vi "QMOLEdll.vi"(8 "error in (no error)":errorcluster, 11 "Inputs":cluster{"qkg":dbl, "xlkg":dbl, "xvkg":dbl}) -> (0 "error out":errorcluster, 3 "Outputs":T1)   [LabVIEW 2016]
doc: "subroutine QMOLEdll(qkg, xlkg, xvkg, qmol, x, y, wliq, wvap, ierr, herr, herr_length\n\nConverts quality and composition on a mass basis to a molar basis\n\nINPUTS:\nqkg -- Quality on mass basis (mass of vapor/total mass) qkg = 0 indicates saturated\n liquid qkg = 1 indicates saturated vapor 0 < qkg < 1 indicates a two-phase state qkg <\n 0 or qkg > 1 are not allowed and will result in warning\nxlkg -- mass composition of liquid phase [array of mass frac]\nxvkg -- mass composition of vapor phase [array of mass frac]\n\nOUTPUTS:\nqmol -- quality on mass basis [mass of vapor/total mass]\nx -- molar composition of liquid phase [array of mol frac]\ny -- molar composition of vapor phase [array of mol frac]\nwliq -- molecular weight of liquid phase [g/mol]\nwvap -- molecular weight of vapor phase [g/mol]\nierr -- error flag: 0 = all inputs within limits, -19 = input q < 0 or > 1\nherr -- error string (character*255 variable if ierr<>0)\nherr_length --length of variable herr (default: 255)"
uses:
  REFPROP.DLL
panel:
  # "REFPROP-QMOLEdll.vi"
  # "void  QMOLEdll(double *qkg, double *xlkg, double *xvkg, double *qmol, double *x, double *y, double *wliq, double *wvap, int32_t *ierr, CStr herr, int32_t herr_length)"
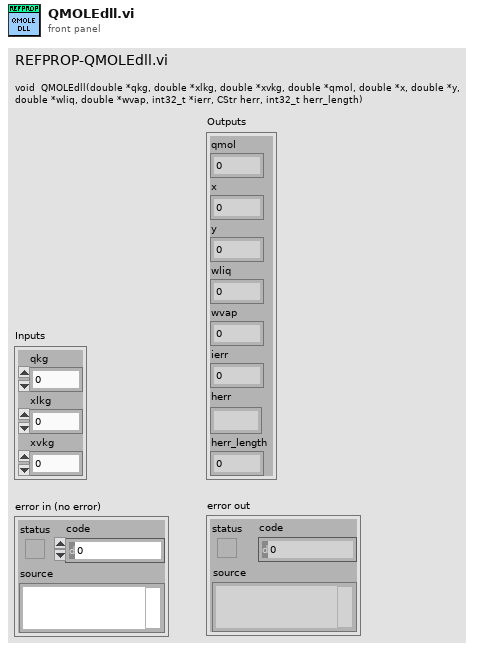
[diagram p1: front panel]
types:
  T1 = cluster{"qmol":dbl, "x":dbl, "y":dbl, "wliq":dbl, "wvap":dbl, "ierr":i32, "herr":string, "herr_length":i32}
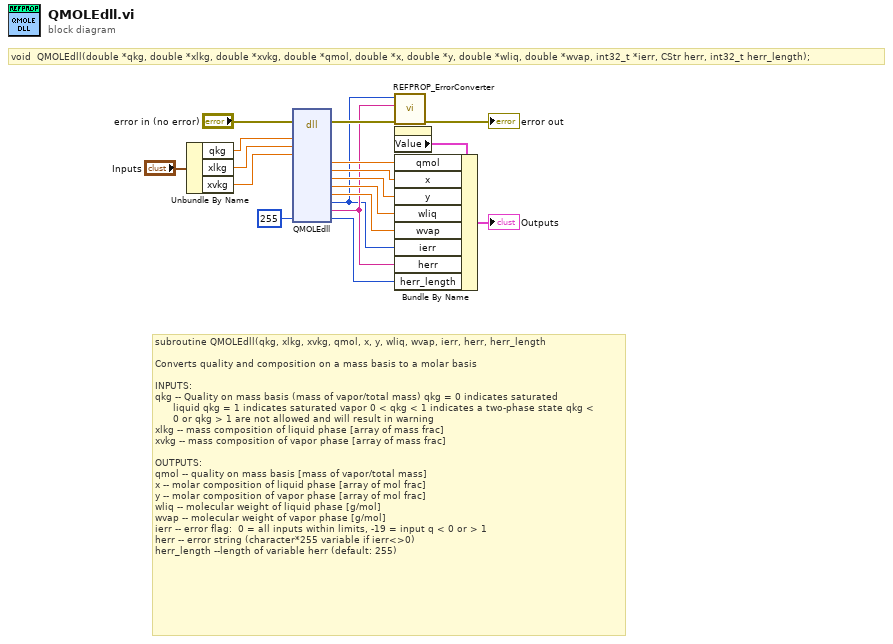
[diagram p0: block diagram]
diagram:
  # "void  QMOLEdll(double *qkg, double *xlkg, double *xvkg, double *qmol, double *x, double *y, double *wliq, double *wvap, int32_t *ierr, CStr herr, int32_t herr_length);"
  # "subroutine QMOLEdll(qkg, xlkg, xvkg, qmol, x, y, wliq, wvap, ierr, herr, herr_length\n\nConverts quality and composition on a mass basis to a molar basis\n\nINPUTS:\nqkg -- Quality on mass basis (mass of vapor/total mass) qkg = 0 indicates saturated\n      liquid qkg = 1 indicates saturated vapor 0 < qkg < 1 indicates a two-phase state qkg <\n      0 or qkg > 1 are not allowed and will result in warning\nxlkg -- mass composition of liquid phase [array of mass frac]\nxvkg -- mass composition of vapor phase [array of mass frac]\n\nOUTPUTS:\nqmol -- quality on mass basis [mass of vapor/total mass]\nx -- molar composition of liquid phase [array of mol frac]\ny -- molar composition of vapor phase [array of mol frac]\nwliq -- molecular weight of liquid phase [g/mol]\nwvap -- molecular weight of vapor phase [g/mol]\nierr -- error flag:  0 = all inputs within limits, -19 = input q < 0 or > 1\nherr -- error string (character*255 variable if ierr<>0)\nherr_length --length of variable herr (default: 255)"
  n1 = Unbundle By Name("Inputs") -> ("qkg"=w13:dbl, "xlkg"=w12:dbl, "xvkg"=w11:dbl)
  n2 = dll-call lib="S:/009 - Testing/02 - Performance Testing/REFPROP/REFPROP.*" fn="QMOLEdll"(error in="error in (no error)", "qkg"=w13, "xlkg"=w12, "xvkg"=w11, "herr_length"=255 ("ln")) -> (error out=w17:errorcluster, "qmol"=w3:dbl, "x"=w4:dbl, "y"=w5:dbl, "wliq"=w6:dbl, "wvap"=w7:dbl, "ierr"=w1:i32, "herr"=w2:string, "herr_length"=w8:i32)  [unwired: 13 in, 1 out]
  n3 = call "REFPROP_ErrorConverter.vi"("error in (no error)"=w17, "Error Message"=w2, "Error Code"=w1) -> ("error out"=→"error out":errorcluster)  [unwired: 8 in]
  n4 = property on="Outputs" class="Clust (strict)"() -> ("Value"=w9:T1)  [unwired: 2 in, 2 out]
  n5 = Bundle By Name(cluster=w9, "qmol"=w3, "x"=w4, "y"=w5, "wliq"=w6, "wvap"=w7, "ierr"=w1, "herr"=w2, "herr_length"=w8) -> (→"Outputs":T1)
